vi "RemoteLogCore.vi"(11 "LoggerMonitorControlData":T1) -> ()   [LabVIEW 2015]
uses:
  LoggerMonitorControlData.ctl
  General/RemoteFiles/connectionData.ctl
panel:
  out "consoleData":string
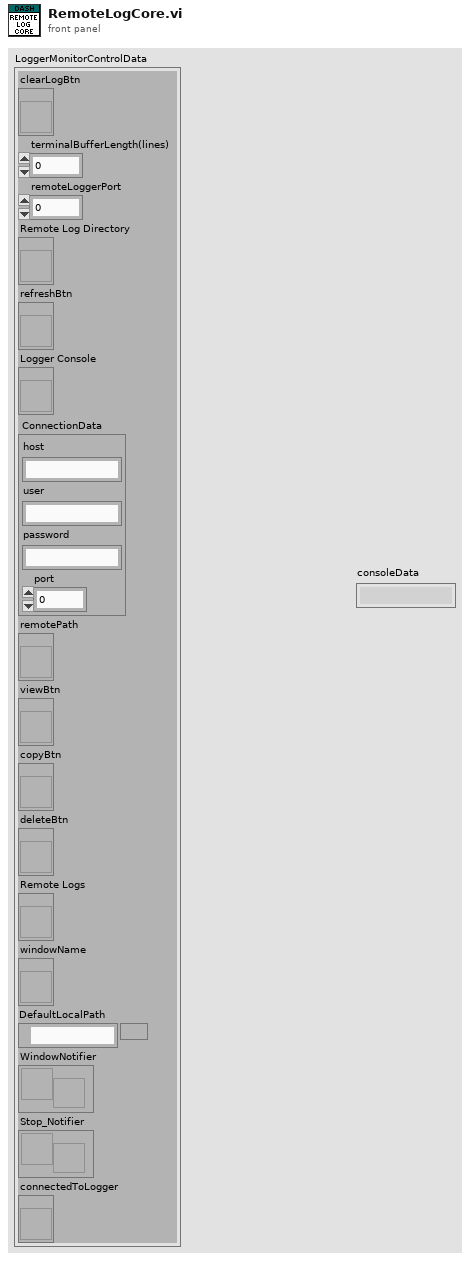
[diagram p1: front panel]
types:
  T1 = typedef "LoggerMonitorControlData.ctl" = cluster{"clearLogBtn":refnum<vi>, "terminalBufferLength(lines)":i32, "remoteLoggerPort":u16, "Remote Log Directory":refnum<vi>, "refreshBtn":refnum<vi>, "Logger Console":refnum<vi>, "ConnectionData":T2, "remotePath":refnum<vi>, "viewBtn":refnum<vi>, "copyBtn":refnum<vi>, "deleteBtn":refnum<vi>, "Remote Logs":refnum<vi>, "windowName":refnum<vi>, "DefaultLocalPath":path, "WindowNotifier":refnum<notifier>, "Stop_Notifier":refnum<notifier>, "connectedToLogger":refnum<vi>}
  T2 = typedef "connectionData.ctl" = cluster{"host":string, "user":string, "password":string, "port":u16}
  T3 = enum16{"Standard", "Buffered", "CRLF", "Immediate"}
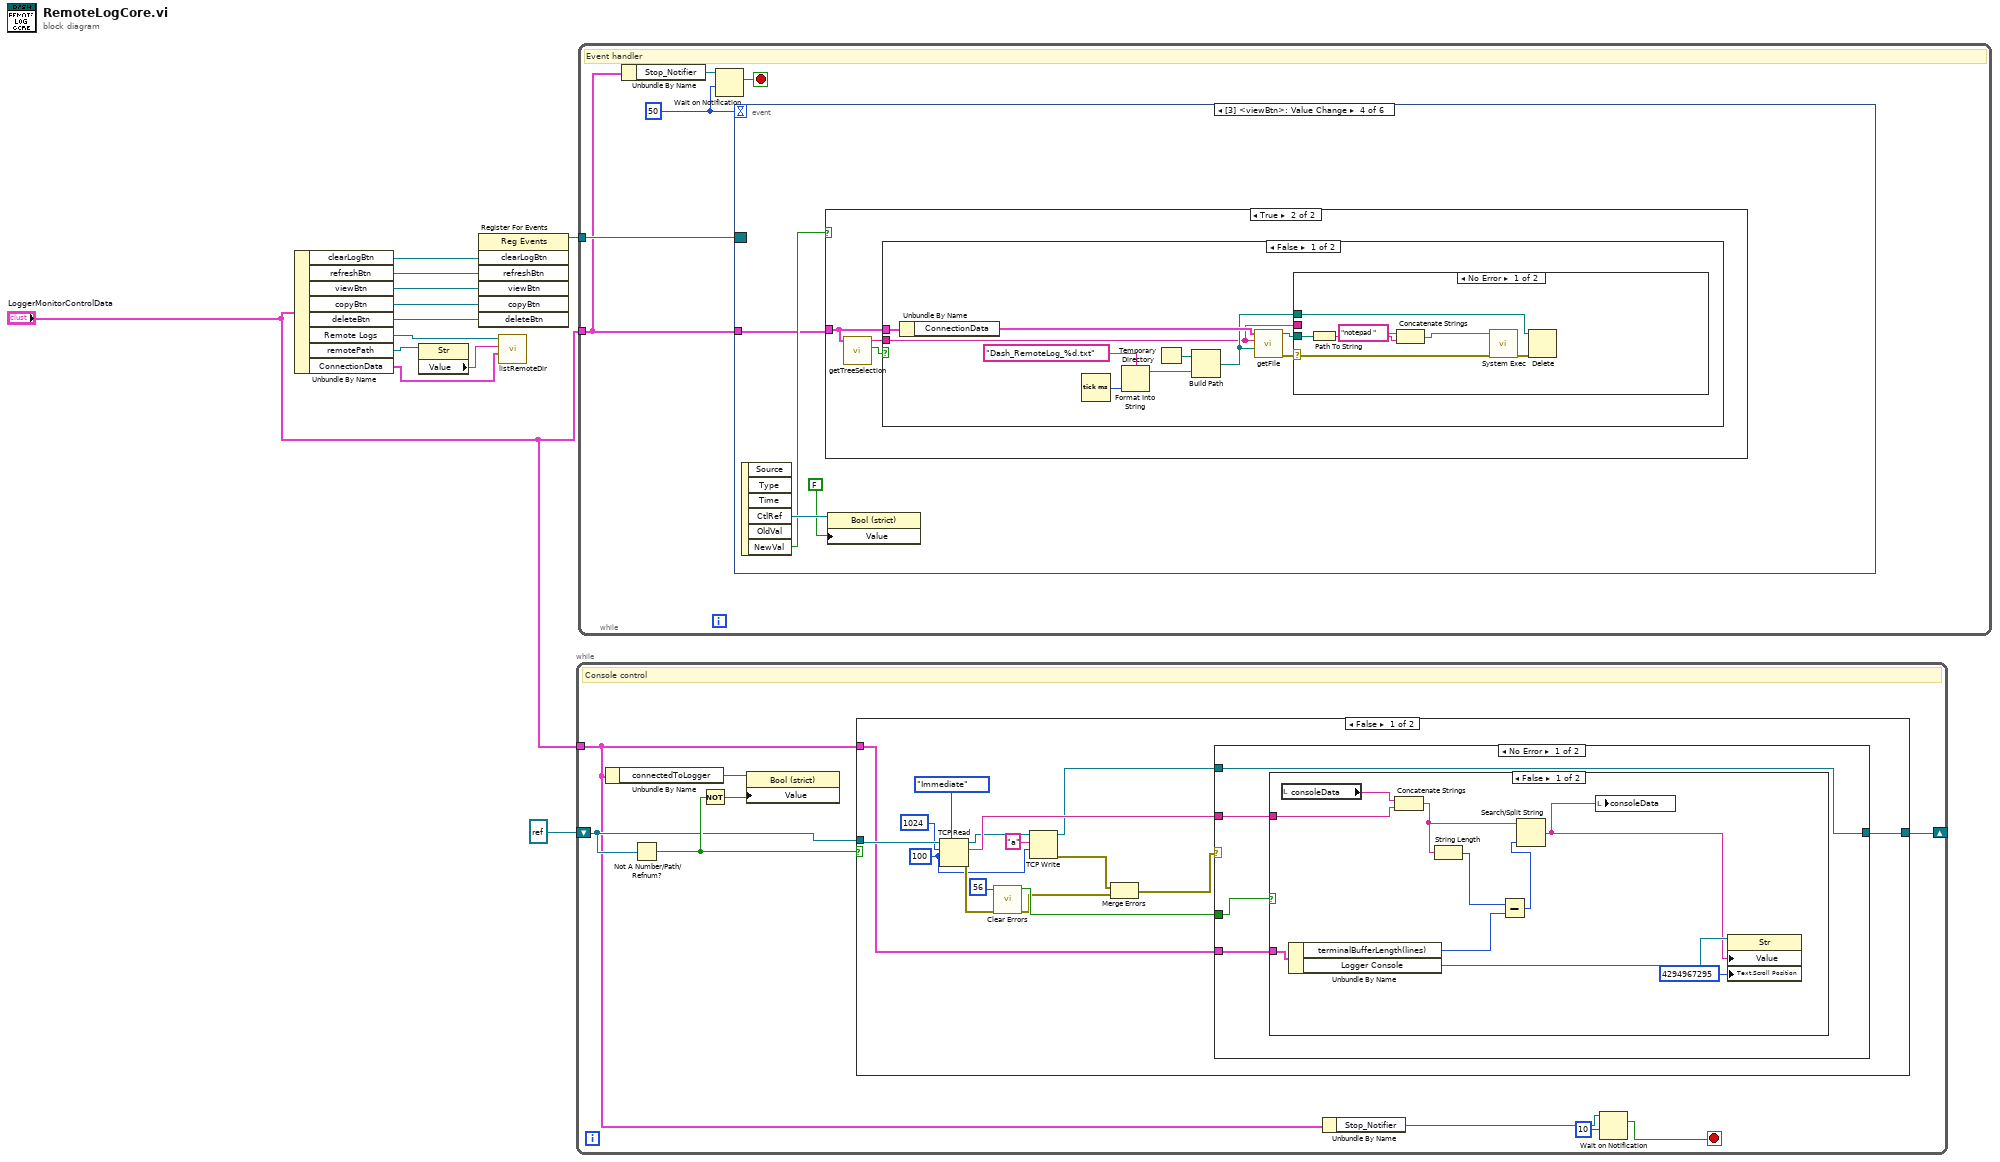
[diagram p0: block diagram]
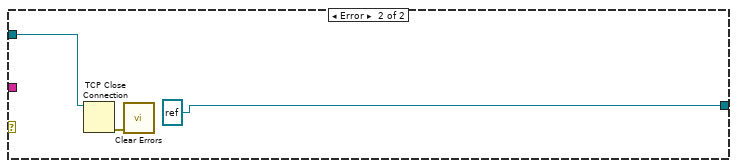
[diagram p3: hidden frame]
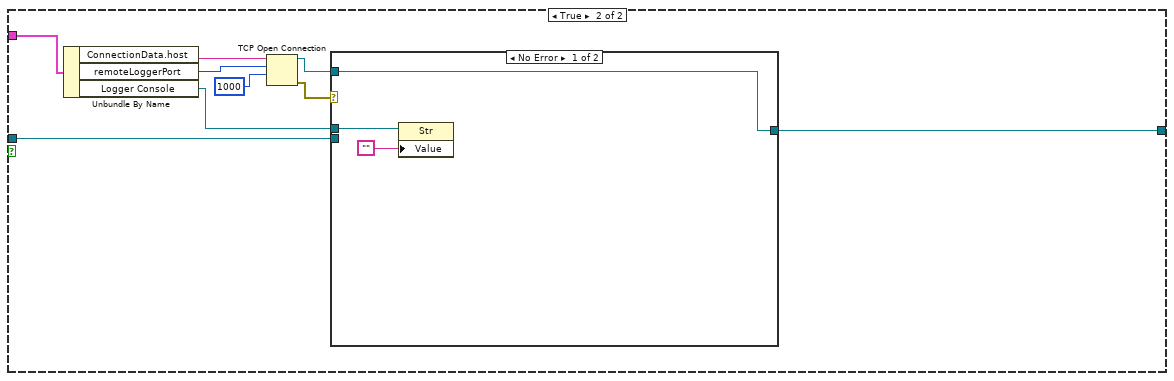
[diagram p4: hidden frame]
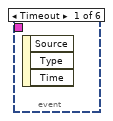
[diagram p6: hidden frame]
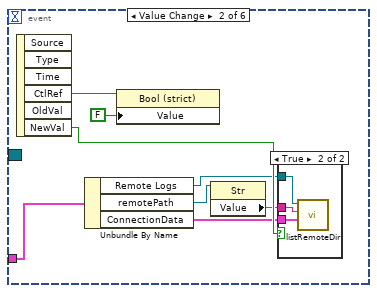
[diagram p7: hidden frame]
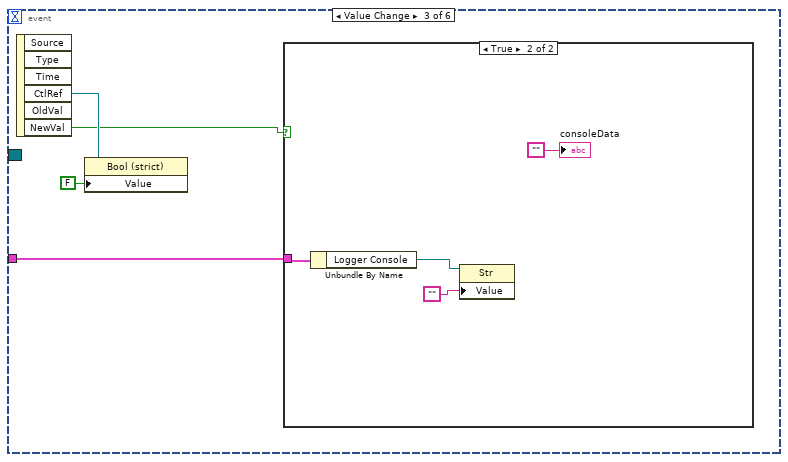
[diagram p9: hidden frame]
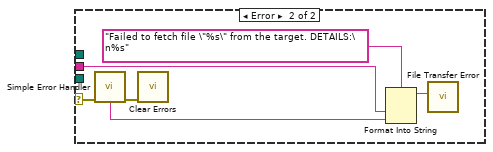
[diagram p12: hidden frame]
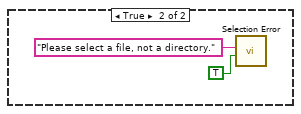
[diagram p13: hidden frame]
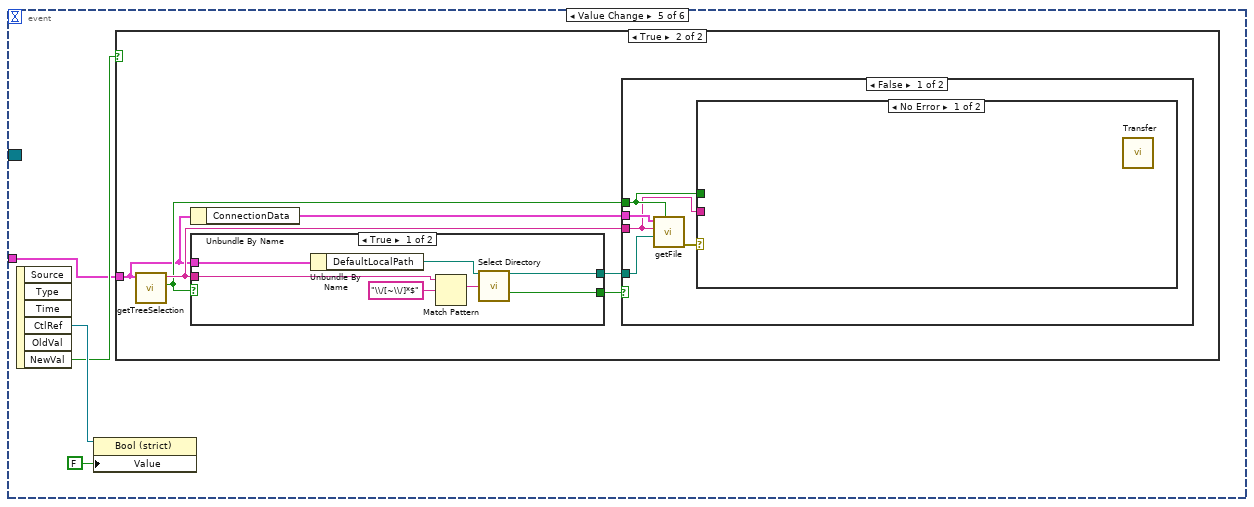
[diagram p14: hidden frame]
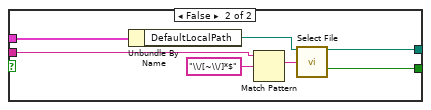
[diagram p16: hidden frame]
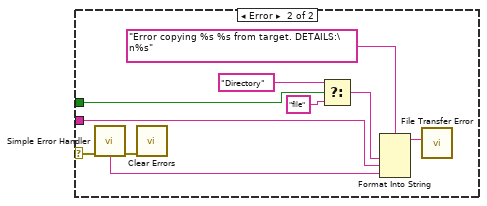
[diagram p17: hidden frame]
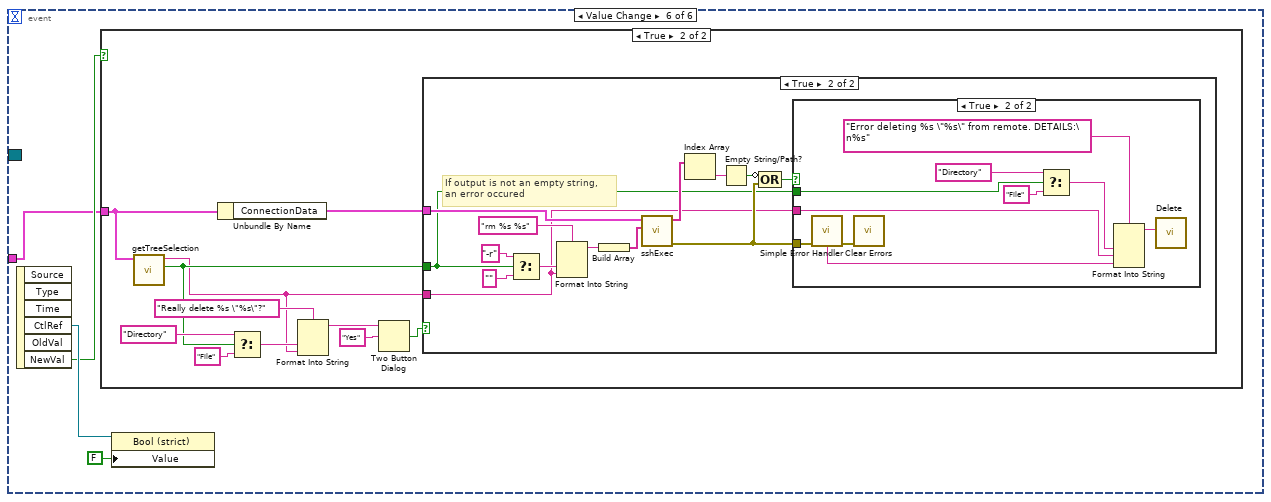
[diagram p19: hidden frame]
diagram:
  n1 = Unbundle By Name("LoggerMonitorControlData") -> ("clearLogBtn"=w12:refnum<vi>, "refreshBtn"=w11:refnum<vi>, "viewBtn"=w10:refnum<vi>, "copyBtn"=w9:refnum<vi>, "deleteBtn"=w8:refnum<vi>, "Remote Logs"=w4:refnum<vi>, "remotePath"=w3:refnum<vi>, "ConnectionData"=w1:T2)
  n2 = property class="Str"(reference=w3) -> ("Value"=w2:string)  [unwired: 1 in, 2 out]
  n3 = register-events(w12, w11, w10, w9, w8) -> (reference out=w7:refnum<event-registration>)  [unwired: 2 in, 1 out]
  n4 = call "listRemoteDir.vi"("ConnectionData"=w1, "remote path"=w2, "TreeControlRefIn"=w4) -> ()  [unwired: 7 in, 2 out]
  n5 = while {
    tunnel: "LoggerMonitorControlData" -> [w16]
    shift-right: [w18] -> _
    shift-left: refnum<k5> refnum ("TCPConnection") -> [w17]
    stop <- w13 stop-if-true
    # "Console control"
    n6 = Unbundle By Name(w16) -> ("connectedToLogger"=w21:refnum<vi>)
    n7 = Not A Number/Path/Refnum?(number/path/refnum=w17) -> (NaN/Path/Refnum?=w19:bool)
    n8 = Not(x=w19) -> (.not. x?=w20:bool)
    n9 = property class="Bool (strict)"(reference=w21, "Value"=w20) -> ()  [unwired: 1 in, 2 out]
    n10 = case shown="False" w19 {
      tunnel: w16 -> [w31 w63]
      tunnel: [w34 w56] -> w18
      tunnel: w17 -> [w37 w55]
      frame False {
        w25 = 100 ("timeout ms (25000)")
        n11 = TCP Read(connection ID=w37, bytes to read=1024, 7:T3."Immediate" ("mode (standard)"), 9:w25) -> (connection ID out=w28:refnum<k5>, data out=w32:string, error out=w36:errorcluster)  [unwired: 1 in]
        n12 = call <vilib>:"Clear Errors.vi"("error in (no error)"=w36, "specific error code to clear (0: all)"=56) -> ("error out"=w24:errorcluster, "specific error cleared?"=w33:bool)  [unwired: 4 in]
        n13 = TCP Write(connection ID=w28, data in="a", 9:w25) -> (connection ID out=w27:refnum<k5>, error out=w23:errorcluster)  [unwired: 1 in, 1 out]
        n14 = Merge Errors(w23, w24) -> (w22:errorcluster)
        n15 = case shown="No Error" w22 {
          tunnel: [w38 refnum<k5> refnum ("TCPConnection")] -> w34
          tunnel: w33 -> [w41 _]
          tunnel: w32 -> [w40 _]
          tunnel: w31 -> [w39 _]
          tunnel: w27 -> [w38 w52]
          frame No Error {
            n16 = case shown="False" w41 {
              tunnel: w40 -> [w42 _]
              tunnel: w39 -> [w51 _]
              frame False {
                n17 = local read "consoleData"() -> (w48:string)
                n18 = Unbundle By Name(w51) -> ("terminalBufferLength(lines)"=w43:i32, "Logger Console"=w50:refnum<vi>)
                n19 = Concatenate Strings(w48, w42) -> (w47:string)
                n20 = String Length(string=w47) -> (length=w44:i32)
                n21 = Subtract(x=w44, y=w43) -> (x-y=w46:i32)
                n22 = Search/Split String(string=w47, offset (0)=w46) -> (match + rest of string=w45:string)  [unwired: 1 in, 2 out]
                n23 = local write "consoleData"(w45) -> ()
                n24 = property class="Str"(reference=w50, "Value"=w45, "Text.Scroll Position"=u32 4294967295) -> ()  [unwired: 1 in, 2 out]
              }
              frame True {
                # "If true, a timeout occured. Just keep going"
              }
            }
          }
          frame Error {
            n25 = TCP Close Connection(connection ID=w52) -> (error out=w54:errorcluster)  [unwired: 2 in, 1 out]
            n26 = call <vilib>:"Clear Errors.vi"("error in (no error)"=w54) -> ()  [unwired: 5 in, 2 out]
          }
        }
      }
      frame True {
        n27 = Unbundle By Name(w63) -> ("ConnectionData.host"=w62:string, "remoteLoggerPort"=w61:u16, "Logger Console"=w57:refnum<vi>)
        n28 = TCP Open Connection(address=w62, remote port or service name=w61, timeout ms (60000)=1000) -> (connection ID=w58:refnum<k5>, error out=w59:errorcluster)  [unwired: 2 in]
        n29 = case shown="No Error" w59 {
          tunnel: w58 -> [w64 _]
          tunnel: w57 -> [w66 _]
          tunnel: [w64 w67] -> w56
          tunnel: w55 -> [_ w67]
          frame No Error {
            n30 = property class="Str"(reference=w66, "Value"="") -> ()  [unwired: 1 in, 2 out]
          }
          frame Error {
          }
        }
      }
    }
    n31 = Unbundle By Name(w16) -> ("Stop_Notifier"=w15:refnum<notifier>)
    n32 = Wait on Notification(notifier=w15, timeout in ms (-1)=10) -> (notification=w13:bool)  [unwired: 2 in, 3 out]
  }
  n33 = while {
    tunnel: w7 -> [w72]
    tunnel: "LoggerMonitorControlData" -> [w70]
    stop <- w71 stop-if-true
    w68 = 50
    # "Event handler"
    n34 = Unbundle By Name(w70) -> ("Stop_Notifier"=w69:refnum<notifier>)
    n35 = Wait on Notification(notifier=w69, timeout in ms (-1)=w68) -> (notification=w71:bool)  [unwired: 2 in, 3 out]
    n36 = event shown="[3] <viewBtn>: Value Change" {
      selector: w72 -> [_ _ _ _ _ _]
      dyn-events: _ -> [_ _ _ _ _ _]
      timeout: w68 -> [_ _ _ _ _ _]
      tunnel: w70 -> [_ w79 w84 w92 w124 w163]
      event Timeout {
        n37 = event-data() -> ()  [unwired: 1 in, 3 out]
      }
      event Value Change {
        n38 = event-data() -> ("CtlRef"=w74:refnum<vi>, "NewVal"=w80:bool)  [unwired: 1 in, 4 out]
        n39 = Unbundle By Name(w79) -> ("Remote Logs"=w78:refnum<vi>, "remotePath"=w77:refnum<vi>, "ConnectionData"=w75:T2)
        n40 = property class="Bool (strict)"(reference=w74, "Value"=FALSE) -> ()  [unwired: 1 in, 2 out]
        n41 = property class="Str"(reference=w77) -> ("Value"=w76:string)  [unwired: 1 in, 2 out]
        n42 = case shown="True" w80 {
          tunnel: w78 -> [_ w83]
          tunnel: w76 -> [_ w82]
          tunnel: w75 -> [_ w81]
          frame False {
          }
          frame True {
            n43 = call "listRemoteDir.vi"("ConnectionData"=w81, "remote path"=w82, "TreeControlRefIn"=w83) -> ()  [unwired: 7 in, 2 out]
          }
        }
      }
      event Value Change {
        n44 = event-data() -> ("CtlRef"=w87:refnum<vi>, "NewVal"=w85:bool)  [unwired: 1 in, 4 out]
        n45 = property class="Bool (strict)"(reference=w87, "Value"=FALSE) -> ()  [unwired: 1 in, 2 out]
        n46 = case shown="True" w85 {
          tunnel: w84 -> [_ w91]
          frame False {
          }
          frame True {
            n47 = Unbundle By Name(w91) -> ("Logger Console"=w90:refnum<vi>)
            n48 = property class="Str"(reference=w90, "Value"="") -> ()  [unwired: 1 in, 2 out]
            "consoleData" <- ""
          }
        }
      }
      event Value Change {
        n49 = event-data() -> ("CtlRef"=w95:refnum<vi>, "NewVal"=w93:bool)  [unwired: 1 in, 4 out]
        n50 = case shown="True" w93 {
          tunnel: w92 -> [_ w96]
          frame False {
          }
          frame True {
            n51 = call "getTreeSelection.vi"("LoggerMonitorControlData"=w96) -> ("isDir?"=w98:bool, "SelectedPath"=w97:string)  [unwired: 8 in, 1 out]
            n52 = case shown="False" w98 {
              tunnel: w97 -> [w99 _]
              tunnel: w96 -> [w108 _]
              frame False {
                n53 = Unbundle By Name(w108) -> ("ConnectionData"=w107:T2)
                n54 = Tick Count (ms)() -> (millisecond timer value=w103:u32)
                n55 = Format Into String(format string="Dash_RemoteLog_%d.txt", w103) -> (resulting string=w104:string)  [unwired: 2 in, 1 out]
                n56 = Temporary Directory() -> (w106:path)
                n57 = Build Path(base path=w106, name or relative path=w104) -> (appended path=w101:path)
                n58 = call "getFile.vi"("local path"=w101, "remote path"=w99, "ConnectionData"=w107) -> ("error out"=w100:errorcluster, "local path out"=w102:path)  [unwired: 7 in]
                n59 = case shown="No Error" w100 {
                  selector: w100 -> [w112 w117]
                  tunnel: w102 -> [w115 _]
                  tunnel: w101 -> [w113 _]
                  tunnel: w99 -> [_ w119]
                  frame No Error {
                    n60 = Path To String(path=w115) -> (string=w111:string)
                    n61 = Concatenate Strings("notepad " ("string"), w111) -> (w109:string)
                    n62 = call <vilib>:"System Exec.vi"("error in (no error)"=w112, "command line"=w109) -> ("error out"=w114:errorcluster)  [unwired: 6 in, 3 out]
                    n63 = Delete(path (use dialog)=w113, error in=w114) -> ()  [unwired: 3 in, 3 out]
                  }
                  frame Error {
                    n64 = call <vilib>:"Simple Error Handler.vi"("error in (no error)"=w117) -> ("error out"=w116:errorcluster, "message"=w118:string)  [unwired: 4 in, 3 out]
                    n65 = call <vilib>:"Clear Errors.vi"("error in (no error)"=w116) -> ()  [unwired: 5 in, 2 out]
                    n66 = Format Into String(format string="Failed to fetch file \"%s\" from the target. DETAILS:\n%s", w119, w118) -> (resulting string=w120:string)  [unwired: 2 in, 1 out]
                    n67 = call "File Transfer Error"("Message"=w120) -> ()  [unwired: 9 in, 2 out]
                  }
                }
              }
              frame True {
                n68 = call "Selection Error"("Enable"=TRUE, "Message"="Please select a file, not a directory.") -> ()  [unwired: 8 in, 2 out]
              }
            }
          }
        }
        n69 = property class="Bool (strict)"(reference=w95, "Value"=FALSE) -> ()  [unwired: 1 in, 2 out]
      }
      event Value Change {
        n70 = event-data() -> ("CtlRef"=w126:refnum<vi>, "NewVal"=w125:bool)  [unwired: 1 in, 4 out]
        n71 = property class="Bool (strict)"(reference=w126, "Value"=FALSE) -> ()  [unwired: 1 in, 2 out]
        n72 = case shown="True" w125 {
          tunnel: w124 -> [_ w131]
          frame False {
          }
          frame True {
            n73 = call "getTreeSelection.vi"("LoggerMonitorControlData"=w131) -> ("isDir?"=w132:bool, "SelectedPath"=w133:string)  [unwired: 8 in, 1 out]
            n74 = Unbundle By Name(w131) -> ("ConnectionData"=w128:T2)
            n75 = case shown="True" w132 {
              tunnel: w133 -> [w139 w146]
              tunnel: w131 -> [w137 w144]
              tunnel: [w135 w142] -> w130
              tunnel: [w134 w141] -> w129
              frame True {
                n76 = Unbundle By Name(w137) -> ("DefaultLocalPath"=w136:path)
                n77 = Match Pattern(string=w139, regular expression="\\/[~\\/]*$") -> (match substring=w138:string)  [unwired: 1 in, 3 out]
                n78 = call "Select Directory"("start path"=w136, "default name"=w138) -> ("selected path"=w134:path, "cancelled"=w135:bool)  [unwired: 10 in, 2 out]
              }
              frame False {
                n79 = Unbundle By Name(w144) -> ("DefaultLocalPath"=w143:path)
                n80 = Match Pattern(string=w146, regular expression="\\/[~\\/]*$") -> (match substring=w145:string)  [unwired: 1 in, 3 out]
                n81 = call "Select File"("start path"=w143, "default name"=w145) -> ("selected path"=w141:path, "cancelled"=w142:bool)  [unwired: 10 in, 2 out]
              }
            }
            n82 = case shown="False" w130 {
              tunnel: w132 -> [w149 _]
              tunnel: w129 -> [w151 _]
              tunnel: w133 -> [w148 _]
              tunnel: w128 -> [w152 _]
              frame False {
                n83 = call "getFile.vi"("isDir?"=w149, "local path"=w151, "remote path"=w148, "ConnectionData"=w152) -> ("error out"=w150:errorcluster)  [unwired: 6 in, 1 out]
                n84 = case shown="No Error" w150 {
                  selector: w150 -> [_ w153]
                  tunnel: w149 -> [_ w155]
                  tunnel: w148 -> [_ w154]
                  frame No Error {
                    n85 = call "Transfer"() -> ()  [unwired: 10 in, 2 out]
                  }
                  frame Error {
                    n86 = call <vilib>:"Simple Error Handler.vi"("error in (no error)"=w153) -> ("error out"=w156:errorcluster, "message"=w157:string)  [unwired: 4 in, 3 out]
                    n87 = call <vilib>:"Clear Errors.vi"("error in (no error)"=w156) -> ()  [unwired: 5 in, 2 out]
                    n88 = Select(t="Directory" ("SelectedPath"), s=w155, f="file") -> (s? t:f=w159:string)
                    n89 = Format Into String(format string="Error copying %s %s from target. DETAILS:\n%s", w159, w154, w157) -> (resulting string=w158:string)  [unwired: 2 in, 1 out]
                    n90 = call "File Transfer Error"("Message"=w158) -> ()  [unwired: 9 in, 2 out]
                  }
                }
              }
              frame True {
              }
            }
          }
        }
      }
      event Value Change {
        n91 = event-data() -> ("CtlRef"=w166:refnum<vi>, "NewVal"=w164:bool)  [unwired: 1 in, 4 out]
        n92 = case shown="True" w164 {
          tunnel: w163 -> [_ w170]
          frame False {
          }
          frame True {
            n93 = call "getTreeSelection.vi"("LoggerMonitorControlData"=w170) -> ("isDir?"=w168:bool, "SelectedPath"=w167:string)  [unwired: 8 in, 1 out]
            n94 = Unbundle By Name(w170) -> ("ConnectionData"=w169:T2)
            n95 = Select(t="Directory", s=w168, f="File") -> (s? t:f=w174:string)
            n96 = Format Into String(format string="Really delete %s \"%s\"?", w174, w167) -> (resulting string=w173:string)  [unwired: 2 in, 1 out]
            n97 = Two Button Dialog(message=w173, 2:"Yes" ("T button name (\"OK\")")) -> (T button?=w171:bool)  [unwired: 1 in]
            n98 = case shown="True" w171 {
              tunnel: w169 -> [_ w185]
              tunnel: w168 -> [_ w179]
              tunnel: w167 -> [_ w178]
              frame False {
              }
              frame True {
                # "If output is not an empty string, \nan error occured"
                n99 = Select(t="-r", s=w179, f="") -> (s? t:f=w188:string)
                n100 = Format Into String(format string="rm %s %s", w188, w178) -> (resulting string=w187:string)  [unwired: 2 in, 1 out]
                n101 = Build Array(w187) -> (w186:string[])
                n102 = call "sshExec.vi"("Commands"=w186, "ConnectionData"=w185) -> ("error out"=w180:errorcluster, "Output"=w184:string[])  [unwired: 8 in]
                n103 = Index Array(array=w184) -> (element=w183:string)  [unwired: 1 in]
                n104 = Empty String/Path?(string/path=w183) -> (empty?=w182:bool)
                n105 = Compound Arithmetic op=OR(invert w182, w180) -> (w181:bool)
                n106 = case shown="True" w181 {
                  tunnel: w180 -> [_ w195]
                  tunnel: w179 -> [_ w198]
                  tunnel: w178 -> [_ w196]
                  frame False {
                    n107 = call "Delete"() -> ()  [unwired: 10 in, 2 out]
                  }
                  frame True {
                    n108 = call <vilib>:"Simple Error Handler.vi"("error in (no error)"=w195) -> ("error out"=w193:errorcluster, "message"=w194:string)  [unwired: 4 in, 3 out]
                    n109 = call <vilib>:"Clear Errors.vi"("error in (no error)"=w193) -> ()  [unwired: 5 in, 2 out]
                    n110 = Select(t="Directory", s=w198, f="File") -> (s? t:f=w197:string)
                    n111 = Format Into String(format string="Error deleting %s \"%s\" from remote. DETAILS:\n%s", w197, w196, w194) -> (resulting string=w192:string)  [unwired: 2 in, 1 out]
                    n112 = call "Delete"("Message"=w192) -> ()  [unwired: 9 in, 2 out]
                  }
                }
              }
            }
          }
        }
        n113 = property class="Bool (strict)"(reference=w166, "Value"=FALSE) -> ()  [unwired: 1 in, 2 out]
      }
    }
  }
